vi "checkErrorInArduinoSerialPort.vi"(8 "error in (no error)":errorcluster) -> (0 "error out":errorcluster, 3 "Porta livre?":bool)   [LabVIEW 2013]
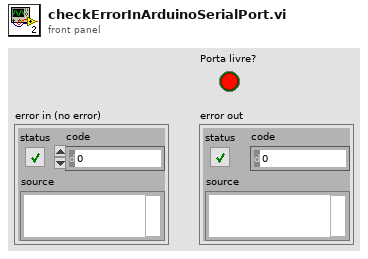
[diagram p1: front panel]
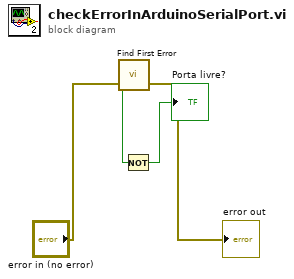
[diagram p0: block diagram]
diagram:
  n1 = call <vilib>:"Find First Error.vi"("error in (no error)"="error in (no error)") -> ("error out"=→"error out":errorcluster, "error?"=w2:bool)  [unwired: 3 in]
  n2 = Not(x=w2) -> (.not. x?=→"Porta livre?":bool)
